vi "Start Calibrate Xtal Dll.vi"(0 "CART TCP Connection In":refnum<k5>, 5 "Need Send Cal Command":u8, 7 "XtalCalGain":u32, 9 "XtalCalCh":u32, 11 "XtalCalFreq":i32) -> (4 "CART TCP Connection Out":refnum<k5>, 6 "StatusIsFalse":i16, 8 "Need More Freq Reporting":i16)   [LabVIEW 2011]
uses:
  WLAN/UUT/QCA/Controls/QCA NART Response Type.ctl
  WLAN/UUT/QCA/NART Constants.vi
panel:
  out "Messages Logged":string[](array[string])
  in  "error in (no error)":errorcluster
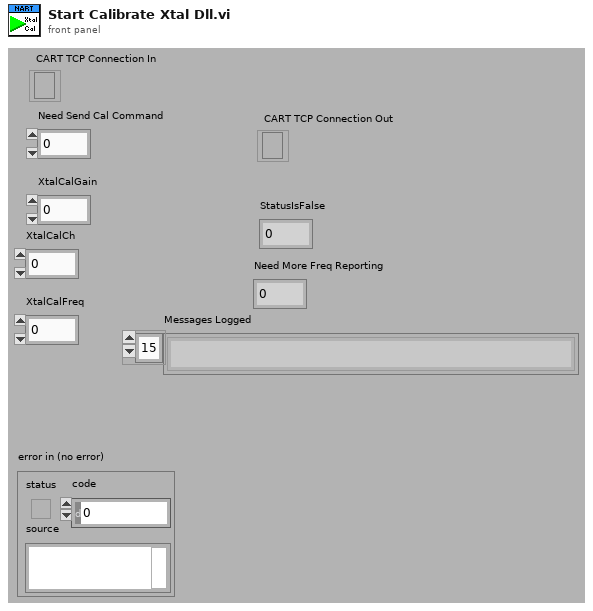
[diagram p1: front panel]
types:
  T1 = typedef "QCA NART Response Type.ctl" = enum16{"DEBUG", "CONTROL", "INFO", "WARNING", "ERROR", "NONE"}
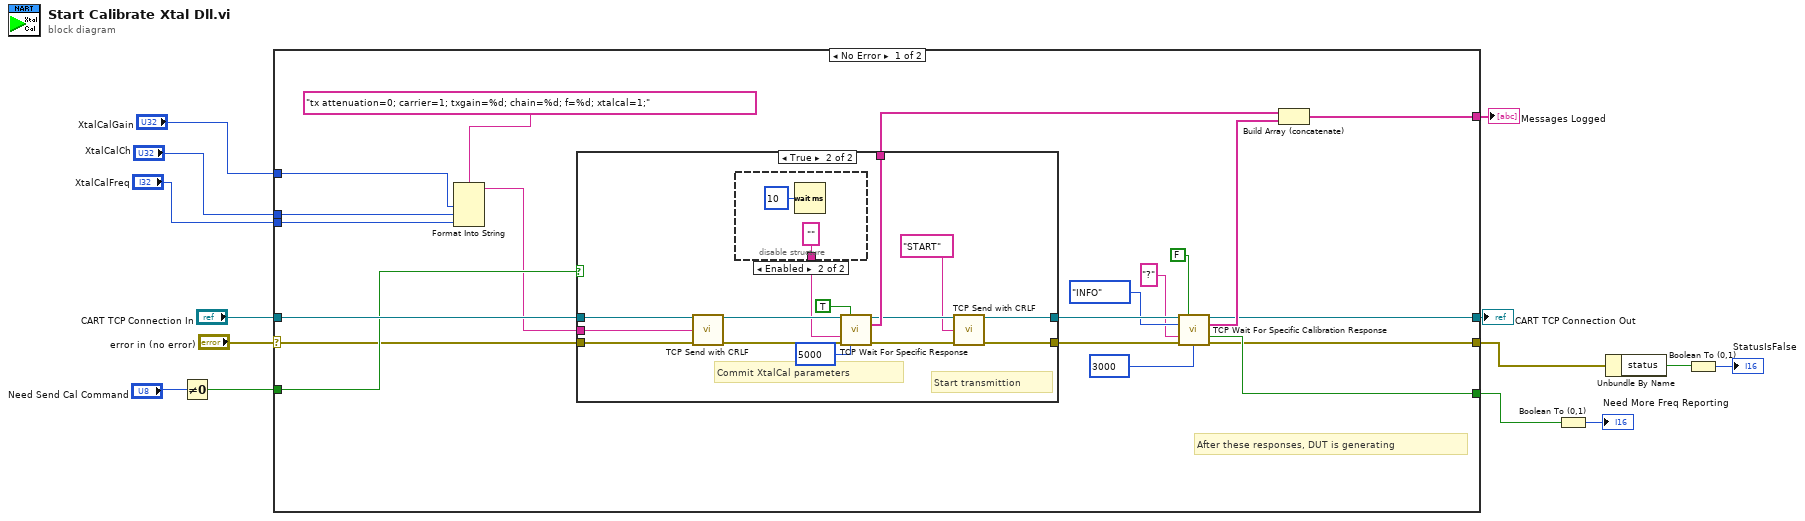
[diagram p0: block diagram]
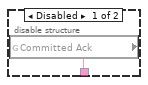
[diagram p3: hidden frame]
diagram:
  n1 = Not Equal To 0?(x="Need Send Cal Command") -> (x != 0?=w3:bool)
  n2 = case shown="No Error" "error in (no error)" {
    selector: "error in (no error)" -> [w21 w55]
    tunnel: [w24 w55] -> w10
    tunnel: "CART TCP Connection In" -> [w34 w54]
    tunnel: [w25 w54] -> w12
    tunnel: [w31 _] -> w11
    tunnel: [w27 _] -> w1
    tunnel: w3 -> [w23 _]
    tunnel: "XtalCalGain" -> [w19 _]
    tunnel: "XtalCalCh" -> [w17 _]
    tunnel: "XtalCalFreq" -> [w16 _]
    frame No Error {
      # "After these responses, DUT is generating"
      n3 = Format Into String(format string="tx attenuation=0; carrier=1; txgain=%d; chain=%d; f=%d; xtalcal=1;" ("Name"), w19, w17, w16) -> (resulting string=w18:string)  [unwired: 2 in, 1 out]
      n4 = case shown="True" w23 {
        tunnel: w34 -> [w36 w50]
        tunnel: [_ w48] -> w33
        tunnel: [w36 w43] -> w30
        tunnel: [w35 w42] -> w29
        tunnel: w21 -> [w35 w38]
        tunnel: w18 -> [_ w37]
        frame False {
        }
        frame True {
          # "Start transmittion"
          # "Commit XtalCal parameters"
          n5 = call "TCP Send with CRLF.vi"("CART TCP Connection"=w50, "data in"=w37, "error IO"=w38) -> ("CART TCP Connection Out"=w47:refnum<k5>, "error out"=w46:errorcluster)  [unwired: 11 in]
          n6 = disable-structure shown="Enabled" {
            disable-tunnel: [w51 "" ("Expected Message Start (\"\":any)")] -> w40
            frame Disabled {
              n7 = global read "NART Constants.vi" "Committed Ack"() -> (w51:string)
            }
            frame Enabled {
              n8 = Wait (ms)(milliseconds to wait=u32 10) -> ()  [unwired: 1 out]
            }
          }
          n9 = call "TCP Wait For Specific Response.vi"("TCP Connection In"=w47, "Next response (t)"=TRUE, "Expected Message Start (\"\":any)"=w40, "error in"=w46, "Timeout (250 ms)"=5000 ("Timeout (100ms)")) -> ("TCP Connection Out"=w44:refnum<k5>, "TCP Messages"=w48:string[], "error out"=w45:errorcluster)  [unwired: 7 in, 1 out]
          n10 = call "TCP Send with CRLF.vi"("CART TCP Connection"=w44, "data in"="START" ("Expected Message Start (\"\":any)"), "error IO"=w45) -> ("CART TCP Connection Out"=w43:refnum<k5>, "error out"=w42:errorcluster)  [unwired: 11 in]
        }
      }
      n11 = call "TCP Wait For Specific Calibration Response.vi"("TCP Connection In"=w30, "Next response (t)"=FALSE, "Expected Type"=QCA_NART_Response_Type."INFO", "Expected Message Start (\"\":any)"="?" ("Expected Message Start (\"\":any)"), "error in"=w29, "Timeout (250 ms)"=3000) -> ("TCP Connection Out"=w25:refnum<k5>, "TCP Messages"=w32:string[], "More Pwr Reporting?"=w27:bool, "error out"=w24:errorcluster)  [unwired: 5 in, 1 out]
      n12 = Build Array (concatenate)(w33, w32) -> (w31:string[])
    }
    frame Error {
    }
  }
  "CART TCP Connection Out" <- w12
  "Messages Logged" <- w11
  n13 = Boolean To (0,1)(Boolean=w1) -> (0, 1=→"Need More Freq Reporting":i16)
  n14 = Unbundle By Name(w10) -> ("status"=w8:bool)
  n15 = Boolean To (0,1)(Boolean=w8) -> (0, 1=→"StatusIsFalse":i16)
